vi "write_sub.vi"(0 "AOUT Array":u16[](array[numeric]), 1 "Motor Val Array":u16[](array[numeric]), 2 "Servo Val Array":u16[](array[numeric]), 8 "OUTTGL":u16, 9 "OUTCLR":u16, 10 "OUTSET":u16, 11 "instance":i32) -> ()   [LabVIEW 2022 SP3]
uses:
  LVLib/SADI_FW3.lvlib
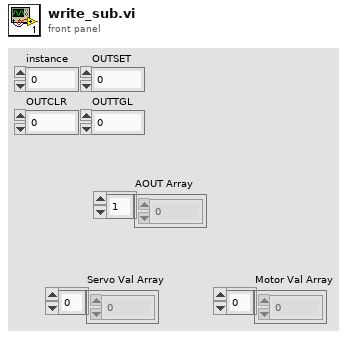
[diagram p1: front panel]
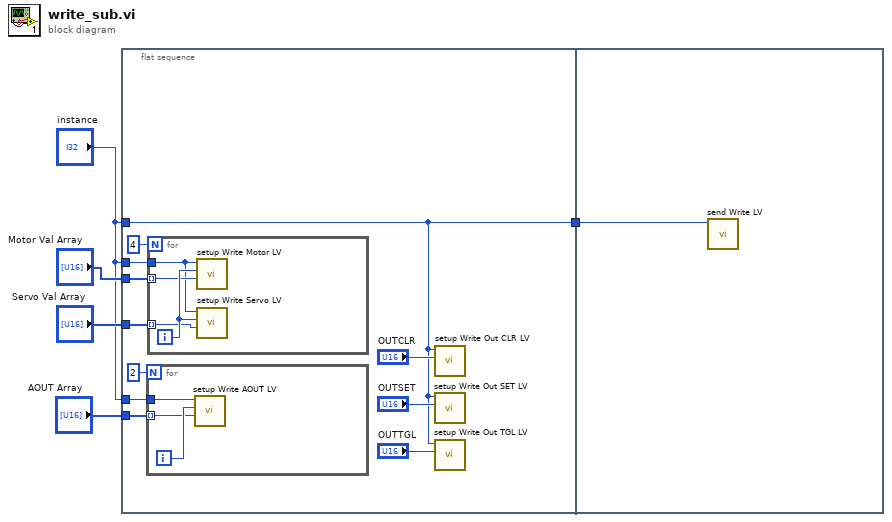
[diagram p0: block diagram]
diagram:
  n1 = flat-sequence {
    tunnel: "AOUT Array" -> [w16]
    tunnel: "instance" -> [w10]
    tunnel: "instance" -> [w7]
    tunnel: "Servo Val Array" -> [w9]
    tunnel: "Motor Val Array" -> [w8]
    tunnel: [w7] -> w2
    tunnel: "instance" -> [w6]
    tunnel: w2 -> [w24]
    frame #0 {
      n2 = for {
        N: 2 -> [_]
        tunnel: w16 -> [w22] mode=indexing
        tunnel: w6 -> [w21]
        i -> [w23]
        n3 = call "setup Write AOUT LV.vi"("AOUT"=w22, "aoutNum"=w23, "instance"=w21) -> ()  [unwired: 9 in]
      }
      n4 = for {
        N: 4 -> [_]
        tunnel: w10 -> [w17]
        tunnel: w9 -> [w19] mode=indexing
        tunnel: w8 -> [w18] mode=indexing
        i -> [w20]
        n5 = call "setup Write Motor LV.vi"("value"=w18, "motorNum"=w20, "instance"=w17) -> ()  [unwired: 9 in]
        n6 = call "setup Write Servo LV.vi"("value"=w19, "servoNum"=w20, "instance"=w17) -> ()  [unwired: 9 in]
      }
      n7 = call "setup Write Out CLR LV.vi"("outMsk"="OUTCLR", "instance"=w7) -> ()  [unwired: 10 in]
      n8 = call "setup Write Out SET LV.vi"("outMsk"="OUTSET", "instance"=w7) -> ()  [unwired: 10 in]
      n9 = call "setup Write Out TGL LV.vi"("outMsk"="OUTTGL", "instance"=w7) -> ()  [unwired: 10 in]
    }
    frame #1 {
      n10 = call "send Write LV.vi"("instance"=w24) -> ()  [unwired: 11 in]
    }
  }
